vi "Coord window-Clear picture.vi"(8 "error in (no error)":errorcluster) -> (0 "error out":errorcluster)   [LabVIEW 2020]
uses:
  Globals/Coord window-Globals.vi
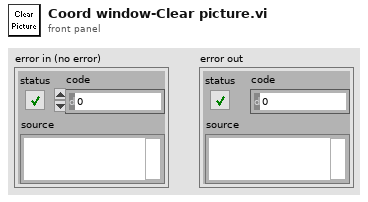
[diagram p1: front panel]
types:
  T1 = cluster{"left":i16, "top":i16, "right":i16, "bottom":i16}
  T2 = typedef "Coordinate list window refs.ctl" = cluster{"Window Name (i.e. Key)":string, "menu reference":refnum<k9>, "VI's reference":refnum<vi>, "Pane 1":refnum<vi>, "Pane 2":refnum<vi>, "Coord Listbox":refnum<vi>, "File name":refnum<vi>, "Picture Map":refnum<vi>, "Stage XYZ Position ind.":refnum<vi>}
  T3 = typedef "LVBoundsTypeDef.ctl" = cluster{"Width":u32, "Height":u32}
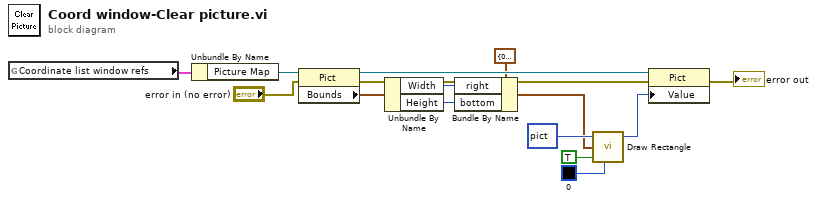
[diagram p0: block diagram]
diagram:
  n1 = global read "Coord window-Globals.vi" "Coordinate list window refs"() -> (w12:T2)
  n2 = Unbundle By Name(w12) -> ("Picture Map"=w9:refnum<vi>)
  n3 = property on="Property Node" class="Pict"(reference=w9, error in="error in (no error)") -> (reference out=w10:refnum<vi>, error out=w14:errorcluster, "Bounds"=w1:T3)
  n4 = Unbundle By Name(w1) -> ("Width"=w7:u32, "Height"=w6:u32)
  n5 = Bundle By Name(cluster=T1 {"left"=0, "top"=0, "right"=30, "bottom"=40} ("rect"), "right"=w7, "bottom"=w6) -> (w2:T1)
  n6 = call <vilib>:"Draw Rectangle.vi"("picture"=picture data[5B] ("2D Picture"), "rect"=w2, "fill?(F)"=TRUE, "color(black)"=u32 0) -> ("new picture"=w11:picture)  [unwired: 5 in]
  n7 = property on="Property Node" class="Pict"(reference=w10, error in=w14, "Value"=w11) -> (error out=→"error out":errorcluster)  [unwired: 1 out]
